vi "Fit Bounds to Size.vi"(10 "size":T1, 11 "FP window bounds in":T2) -> (3 "FP window bounds out":T2)   [LabVIEW 2010, in "NI_SE_Front Panel Layout.lvlib"]
uses:
  NI_SE_Front Panel Layout.lvlib
  <vilib>/Utility/miscctls.llb/LVRectTypeDef.ctl
  <vilib>/Utility/miscctls.llb/LVPointTypeDef.ctl
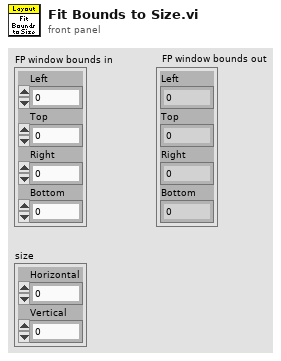
[diagram p1: front panel]
types:
  T1 = typedef "LVPointTypeDef.ctl" = cluster{"Horizontal":i16, "Vertical":i16}
  T2 = typedef "LVRectTypeDef.ctl" = cluster{"Left":i16, "Top":i16, "Right":i16, "Bottom":i16}
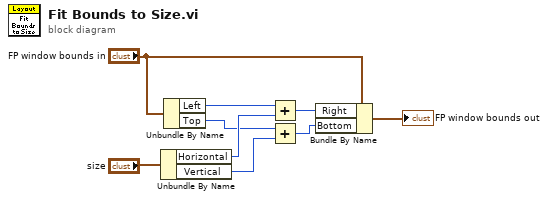
[diagram p0: block diagram]
diagram:
  n1 = Unbundle By Name("size") -> ("Horizontal"=w5:i16, "Vertical"=w2:i16)
  n2 = Unbundle By Name("FP window bounds in") -> ("Left"=w6:i16, "Top"=w3:i16)
  n3 = Add(x=w6, y=w5) -> (x+y=w4:i16)
  n4 = Add(x=w3, y=w2) -> (x+y=w1:i16)
  n5 = Bundle By Name(cluster="FP window bounds in", "Right"=w4, "Bottom"=w1) -> (→"FP window bounds out":T2)
